vi "CreateActionQueues.vi"(8 "Error In":errorcluster) -> (0 "Error Out":errorcluster, 3 "Action Queues":T1)   [LabVIEW 2012]
uses:
  ActionQueues.ctl
  UIActionQueueElement.ctl
  UIAction.ctl
  HardwareActionQueueElement.ctl
  HardwareAction.ctl
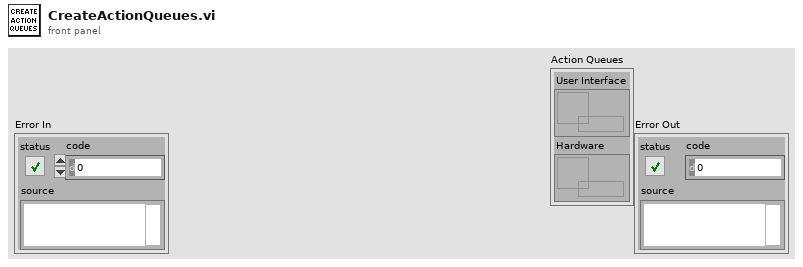
[diagram p1: front panel]
types:
  T1 = typedef "ActionQueues.ctl" = cluster{"User Interface":refnum<queue>, "Hardware":refnum<queue>}
  T2 = typedef "HardwareActionQueueElement.ctl" = cluster{"Action":T3, "Data":variant}
  T3 = typedef "HardwareAction.ctl" = enum16{"Initialize", "Start", "Stop", "Error", "Shutdown"}
  T4 = typedef "UIActionQueueElement.ctl" = cluster{"Action":T5, "Data":variant}
  T5 = typedef "UIAction.ctl" = enum16{"Initialize", "Configure Trigger", "Configure Scan", "Configure Memory", "Configure Slot 1", "Open", "Save", "Reset", "Start", "Started", "Stop", "Stopped", "Shutdown"}
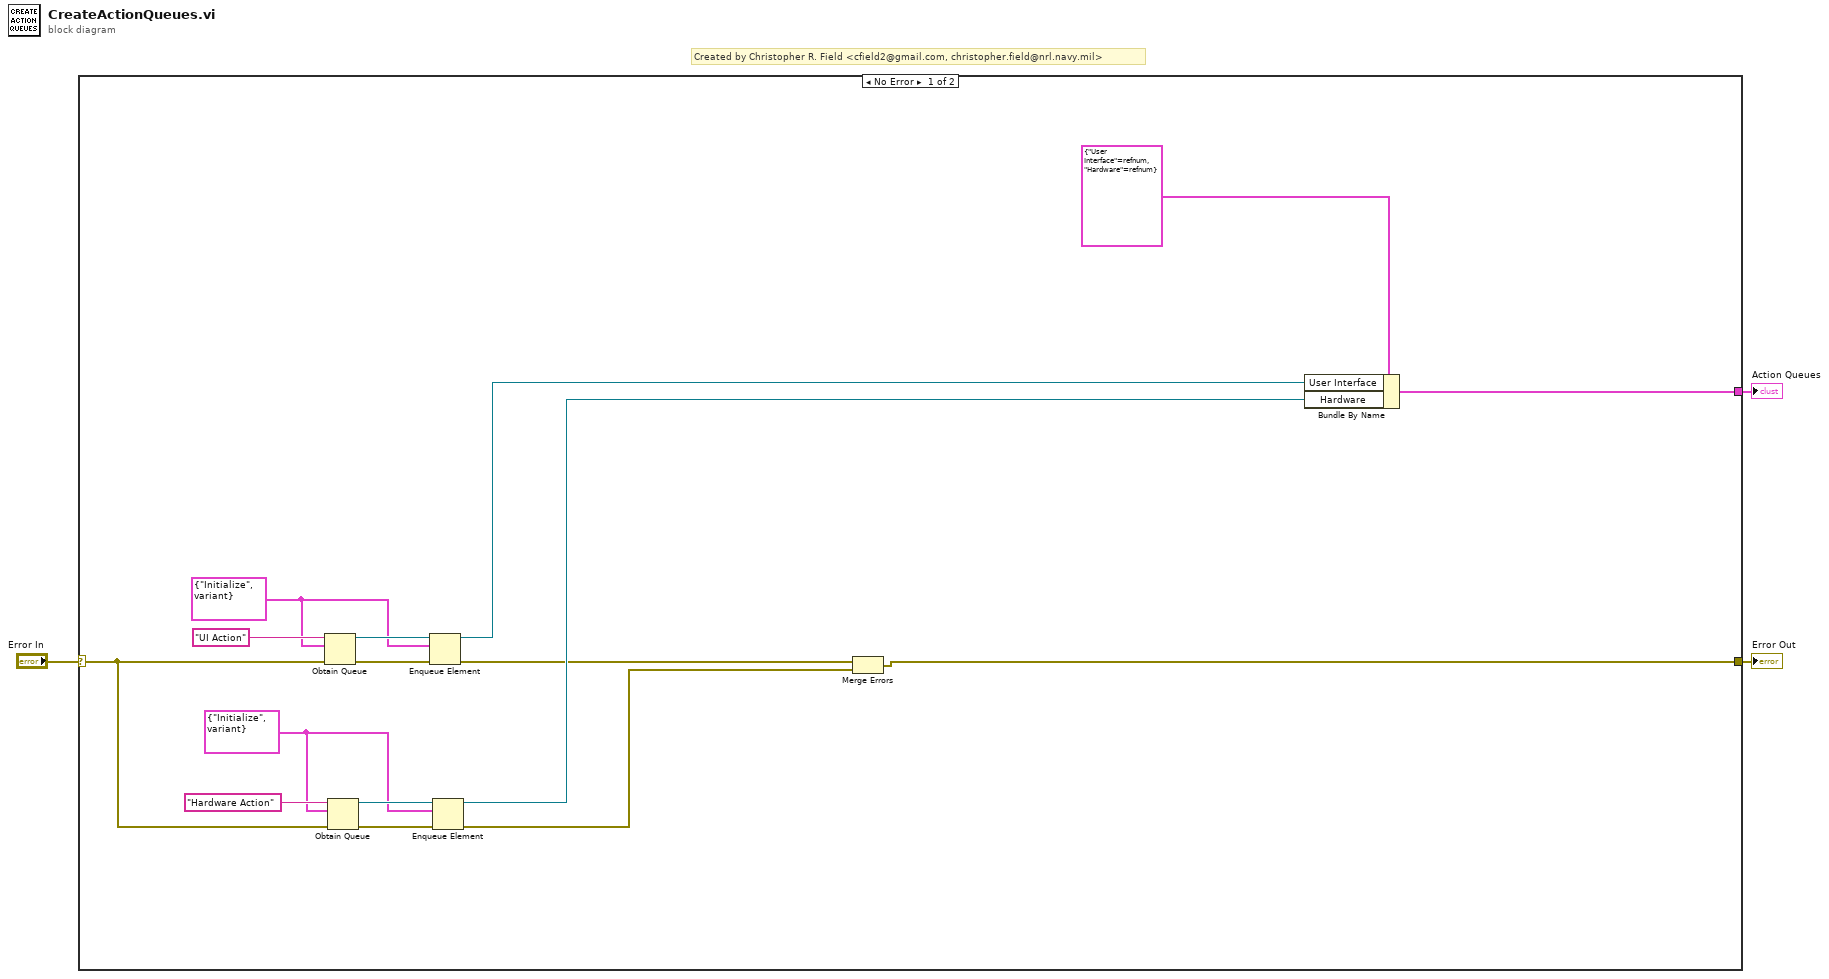
[diagram p0: block diagram]
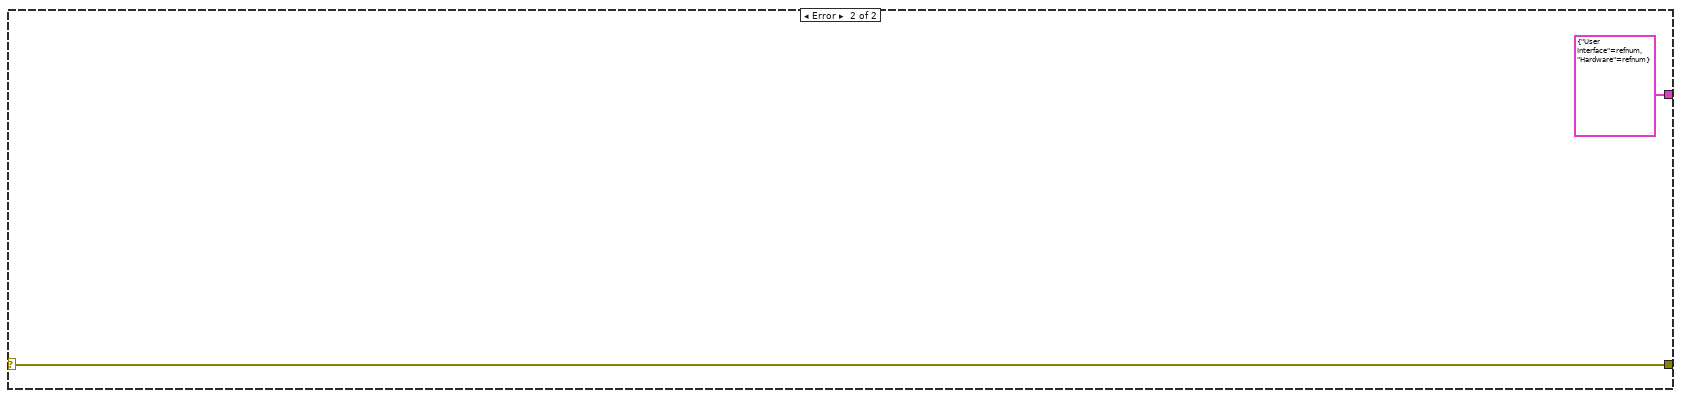
[diagram p2: hidden frame]
diagram:
  # "Created by Christopher R. Field <cfield2@gmail.com, christopher.field@nrl.navy.mil>"
  n1 = case shown="No Error" "Error In" {
    selector: "Error In" -> [w10 w21]
    tunnel: [w5 w21] -> w1
    tunnel: [w13 T1 {"User Interface"=refnum, "Hardware"=refnum} ("Action Queues")] -> w2
    frame No Error {
      w4 = T2 {"Action"=enum."Initialize", "Data"=variant} ("Hardware Action Queue Element")
      w16 = T4 {"Action"=enum."Initialize", "Data"=variant} ("UI Action Queue Element")
      n2 = Obtain Queue(name (unnamed)="UI Action", element data type=w16, error in (no error)=w10) -> (queue out=w18:refnum<queue>, error out=w17:errorcluster)  [unwired: 2 in, 1 out]
      n3 = Obtain Queue(name (unnamed)="Hardware Action", element data type=w4, error in (no error)=w10) -> (queue out=w12:refnum<queue>, error out=w11:errorcluster)  [unwired: 2 in, 1 out]
      n4 = Enqueue Element(queue=w18, element=w16, error in (no error)=w17) -> (queue out=w14:refnum<queue>, error out=w7:errorcluster)  [unwired: 1 in, 1 out]
      n5 = Enqueue Element(queue=w12, element=w4, error in (no error)=w11) -> (queue out=w8:refnum<queue>, error out=w6:errorcluster)  [unwired: 1 in, 1 out]
      n6 = Merge Errors(w7, w6) -> (w5:errorcluster)
      n7 = Bundle By Name(cluster=T1 {"User Interface"=refnum, "Hardware"=refnum} ("Action Queues"), "User Interface"=w14, "Hardware"=w8) -> (w13:T1)
    }
    frame Error {
    }
  }
  "Action Queues" <- w2
  "Error Out" <- w1
